vi "Wait Until Digital Count.vi"(0 "Device ID":T4(ring), 2 "Wait Until":T2(ring), 5 "Module":T1(ring), 7 "Digital_Input":T3(ring), 9 "Final Count":u32=1, 11 "error in":errorcluster, 13 "Time Out (10)":dbl=10.0) -> (4 "Device ID Out":T4(ring), 15 "error out":errorcluster)   [LabVIEW 2010]
doc: "This VI waits until a specified number of user-defined digital edges are read."
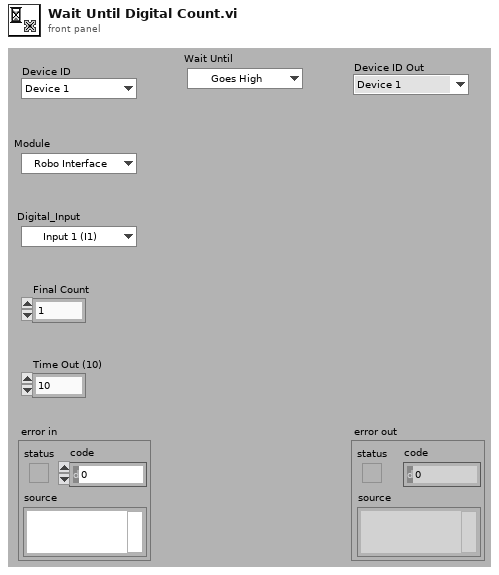
[diagram p1: front panel]
types:
  T1 = enum8{"Robo Interface", "Extension 1", "Extension 2", "Extension 3"}
  T2 = enum8{"Goes High", "Goes Low", "Goes High or Low"}
  T3 = enum8{"Input 1 (I1)", "Input 2 (I2)", "Input 3 (I3)", "Input 4 (I4)", "Input 5 (I5)", "Input 6 (I6)", "Input 7 (I7)", "Input 8 (I8)"}
  T4 = enum16{"Device 1", "Device 2", "Device 3", "Device 4", "Device 5", "Device 6", "Device 7", "Device 8"}
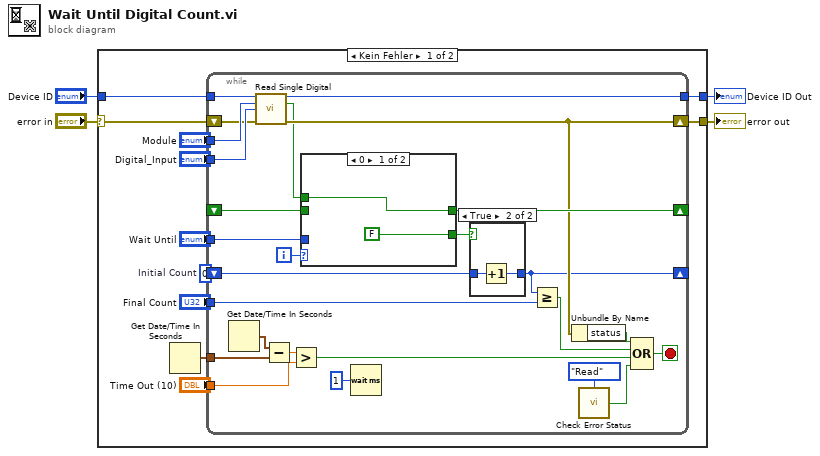
[diagram p0: block diagram]
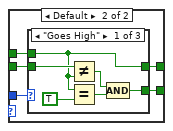
[diagram p3: hidden frame]
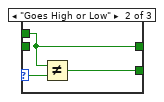
[diagram p4: hidden frame]
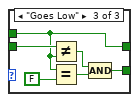
[diagram p5: hidden frame]
diagram:
  n1 = case shown="Kein Fehler" "error in" {
    selector: "error in" -> [w8 w68]
    tunnel: [w7 w68] -> w3
    tunnel: "Device ID" -> [w10 w67]
    tunnel: [w9 w67] -> w1
    frame No Error {
      w6 = u32 0  # Initial Count
      n2 = Get Date/Time In Seconds() -> (seconds since 1Jan1904=w14:timestamp)
      n3 = while {
        tunnel: "Wait Until" -> [w41]
        shift-right: [w35] -> _
        shift-left: _ -> [w34]
        tunnel: w14 -> [w39]
        tunnel: "Time Out (10)" -> [w37]
        tunnel: w10 -> [w30]
        tunnel: "Module" -> [w29]
        tunnel: "Digital_Input" -> [w28]
        tunnel: [w27] -> w9
        shift-right: [w25] -> w7
        shift-left: w8 -> [w26]
        shift-right: [w19] -> _
        shift-left: w6 -> [w22]
        tunnel: "Final Count" -> [w20]
        i -> [w36]
        stop <- w32 stop-if-true
        n4 = Get Date/Time In Seconds() -> (seconds since 1Jan1904=w40:timestamp)
        n5 = call "Read Single Digital.vi"("Device ID"=w30, "Module"=w29, "Digital_Input"=w28, "error in"=w26) -> ("Device ID Out"=w27:T4, "Value"=w18:bool, "error out"=w25:errorcluster)  [unwired: 9 out]
        n6 = Subtract(x=w40, y=w39) -> (x-y=w38:dbl)
        n7 = Greater?(x=w38, y=w37) -> (0:w33:bool)
        n8 = case shown="0" w36 {
          tunnel: w41 -> [_ w51]
          tunnel: [w45 w49] -> w35
          tunnel: w34 -> [_ w50]
          tunnel: [FALSE w48] -> w23
          tunnel: w18 -> [w45 w47]
          frame 0 {
          }
          frame Default {
            n9 = case shown="\"Goes High\"" w51 {
              tunnel: w50 -> [w57 w60 w63]
              tunnel: [w52 w58 w61] -> w49
              tunnel: [w53 w59 w62] -> w48
              tunnel: w47 -> [w52 w58 w61]
              frame "Goes High" {
                n10 = Not Equal?(x=w57, y=w52) -> (x != y?=w55:bool)
                n11 = Equal?(x=w52, y=TRUE) -> (x = y?=w54:bool)
                n12 = Compound Arithmetic op=AND(w55, w54) -> (w53:bool)
              }
              frame "Goes High or Low" {
                n13 = Not Equal?(x=w58, y=w60) -> (x != y?=w59:bool)
              }
              frame "Goes Low" {
                n14 = Not Equal?(x=w63, y=w61) -> (x != y?=w65:bool)
                n15 = Equal?(x=w61, y=FALSE) -> (x = y?=w64:bool)
                n16 = Compound Arithmetic op=AND(w65, w64) -> (w62:bool)
              }
            }
          }
        }
        n17 = Wait (ms)(milliseconds to wait=u32 1) -> ()  [unwired: 1 out]
        n18 = case shown="TRUE" w23 {
          tunnel: [w42 w43] -> w19
          tunnel: w22 -> [w42 w44]
          frame False {
          }
          frame True {
            n19 = Increment(x=w44) -> (x+1=w43:u32)
          }
        }
        n20 = Greater Or Equal?(x=w19, y=w20) -> (x >= y?=w21:bool)
        n21 = Unbundle By Name(w25) -> ("status"=w24:bool)
        n22 = call "Check Error Status.vi"("Action (Write)"=enum16{"Write", "Read"}."Read") -> ("Error?"=w16:bool)  [unwired: 2 in, 12 out]
        n23 = Compound Arithmetic op=OR(w24, w21, w33, w16) -> (w32:bool)
      }
    }
    frame Error {
    }
  }
  "error out" <- w3
  "Device ID Out" <- w1
